vi "DB Tools Format Datetime String (Time Stamp).vi"(1 "time stamp":timestamp) -> (0 "date/time string":string)   [LabVIEW 2012, in "NI_Database_API_64.lvlib"]
doc: "Returns a string containing the formatted date and time, and identifies the string as a date/time string so other VIs can interpret this string. Wire data to the input of this VI to determine the polymorphic instance to use or manually select the instance."
uses:
  NI_Database_API_64.lvlib
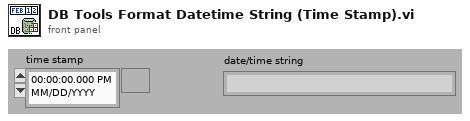
[diagram p1: front panel]
types:
  T1 = typedef "LVDateTimeRec.ctl" = cluster{"fractional second":dbl, "second":i32, "minute":i32, "hour":i32, "day of month":i32, "month":i32, "year":i32, "day of week":i32, "day of year":i32, "DST":i32}
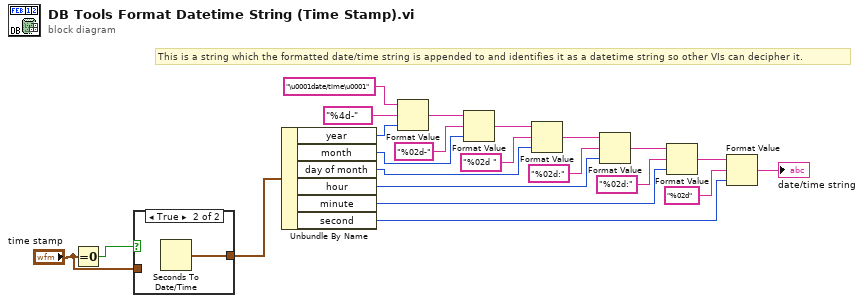
[diagram p0: block diagram]
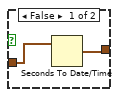
[diagram p2: hidden frame]
diagram:
  # "This is a string which the formatted date/time string is appended to and identifies it as a datetime string so other VIs can decipher it."
  n1 = Equal To 0?(x="time stamp") -> (x = 0?=w2:bool)
  n2 = case shown="True" w2 {
    tunnel: [w23 w25] -> w3
    tunnel: "time stamp" -> [w24 _]
    frame False {
      n3 = Seconds To Date/Time(time stamp (now)=w24) -> (date time rec=w23:T1)  [unwired: 1 in]
    }
    frame True {
      n4 = Seconds To Date/Time() -> (date time rec=w25:T1)  [unwired: 2 in]
    }
  }
  n5 = Unbundle By Name(w3) -> ("year"=w10:i32, "month"=w9:i32, "day of month"=w8:i32, "hour"=w22:i32, "minute"=w19:i32, "second"=w18:i32)
  n6 = Format Value(string ("")="\u0001date/time\u0001", format string="%4d-", value (0)=w10) -> (output string=w13:string)
  n7 = Format Value(string ("")=w13, format string="%02d-", value (0)=w9) -> (output string=w12:string)
  n8 = Format Value(string ("")=w12, format string="%02d ", value (0)=w8) -> (output string=w11:string)
  n9 = Format Value(string ("")=w11, format string="%02d:", value (0)=w22) -> (output string=w21:string)
  n10 = Format Value(string ("")=w21, format string="%02d:", value (0)=w19) -> (output string=w20:string)
  n11 = Format Value(string ("")=w20, format string="%02d", value (0)=w18) -> (output string=→"date/time string":string)
